vi "FTW-Example-Actors.vi"() -> ()   [LabVIEW 2013]
uses:
  source/actor/Connector/FTW-ActorConnector.lvclass
  source/actor/Ether/FTW-Ether.lvclass
panel:
  out "Response Body":string
  out "Instance Inbox Address":string
  out "Initialized Response":string
  out "Timed out?":bool
  out "Ping Response":string
  in  "FTW Ether Configuration":string="{\n  \"ApplicationName\": \"Actor Example\",\n  \"ApplicationVersion\": \"0.1.0-1\",\n  \"LoggerAddress\": \"inproc://*\",\n  \"LoggerName\": \"ActorExample\",\n  \"LoggerDirectory\": \"[UserDesktop]\\\\Logs\",\n  \"LoggerDiskThrashDelay\": 200\n}"
  in  "Actor 1 Configuration":string="{\n  \"Identity\": \"FeatherweightActorExample\",\n  \"InboxAddress\": \"inproc://*\",\n  \"LoggerAddress\": \"\",\n  \"DebugEnableInboxLogging\": false,\n  \"DebugEnableJobLogging\": false,\n  \"DebugShowPanel\": false\n}"
  out "error out":errorcluster
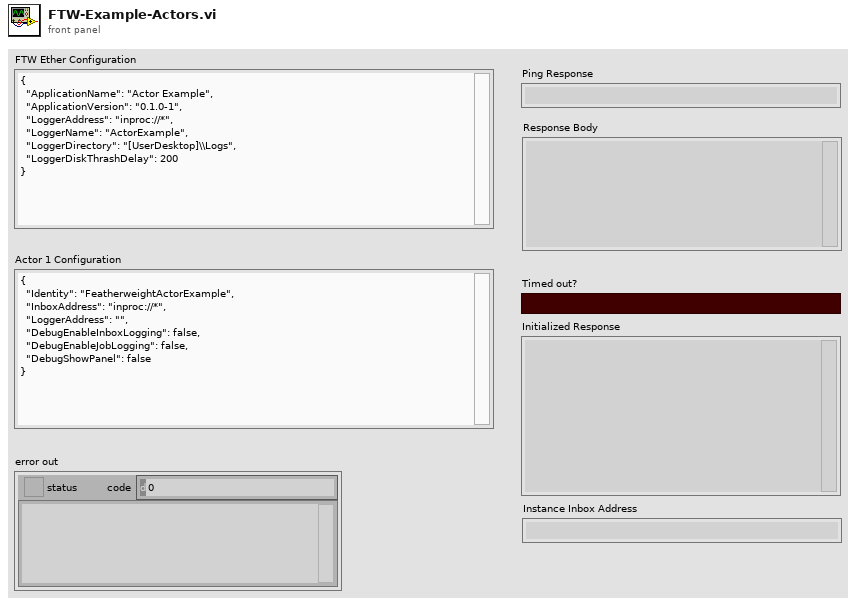
[diagram p1: front panel]
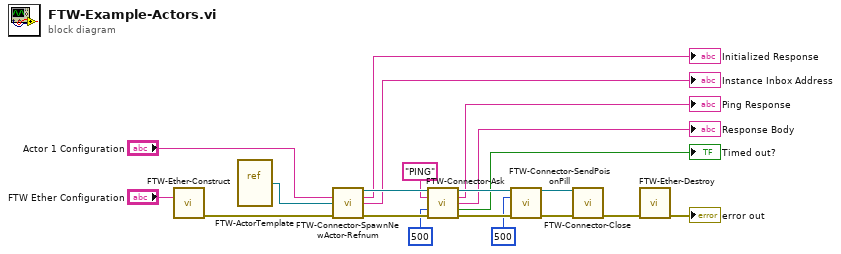
[diagram p0: block diagram]
diagram:
  n1 = call "FTW-Ether-Construct.vi"("FTW Ether Configuration"="FTW Ether Configuration") -> ("error out"=w17:errorcluster)  [unwired: 14 in]
  n2 = vi-ref "FTW-ActorTemplate.vi"() -> (w1:refnum<vi>)
  n3 = call "FTW-Connector-SpawnNewActor-Refnum.vi"("Configuration"="Actor 1 Configuration", "Actor VI Refnum"=w1, "error in"=w17) -> ("FTW Actor Connector"=w20:refnum<class "FTW-ActorConnector.lvclass">, "Initialized Response"=→"Initialized Response":string, "Instance Inbox Address"=→"Instance Inbox Address":string, "error out"=w9:errorcluster)  [unwired: 9 in]
  n4 = call "FTW-Connector-Ask.vi"("FTW Actor Connector"=w20, "Request Header"="PING", "Timeout"=500, "error in"=w9) -> ("FTW Actor Connector out"=w19:refnum<class "FTW-ActorConnector.lvclass">, "Response Header"=→"Ping Response":string, "Response Body"=→"Response Body":string, "Timed out?"=→"Timed out?":bool, "error out"=w7:errorcluster)  [unwired: 5 in, 2 out]
  n5 = call-dynamic "FTW-Connector-SendPoisonPill.vi"("FTW Actor Connector"=w19, "Timeout"=500, "error in"=w7) -> ("FTW Actor Connector out"=w6:refnum<class "FTW-ActorConnector.lvclass">, "error out"=w5:errorcluster)  [unwired: 8 in, 3 out]
  n6 = call-dynamic "FTW-Connector-Close.vi"("FTW Actor Connector"=w6, "error in"=w5) -> ("error out"=w13:errorcluster)  [unwired: 13 in]
  n7 = call "FTW-Ether-Destroy.vi"("error in"=w13) -> ("error out"=→"error out":errorcluster)  [unwired: 14 in]
